vi "Send Software Trigger.vi"(8 "error in (no error)":errorcluster, 11 "VISA resource name":refnum<visa-resource-name>) -> (0 "error out":errorcluster, 3 "VISA resource name out":refnum<visa-resource-name>)   [LabVIEW 2015, in "Agilent 3352X Series.lvlib"]
doc: "Sends a software bus trigger to the instrument. You can use software bus triggers to trigger a frequency sweep. You must first set Trigger Source in the Configure Trigger VI to Software. \n\n<B>Note</B>:\n(1) Use this VI only with other low-level VIs. The high-level VIs automatically incorporate this functionality. \n(2) This VI does not check the instrument status. If you want to check the instrument status, call the Error Query VI at the conclusion of your sweep operation."
uses:
  Agilent 3352X Series.lvlib
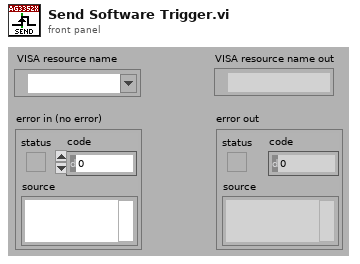
[diagram p1: front panel]
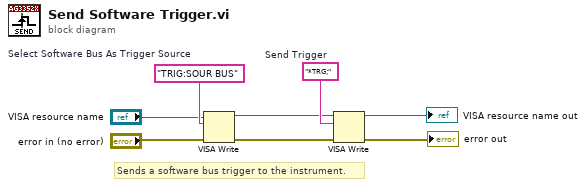
[diagram p0: block diagram]
diagram:
  w5 = "TRIG:SOUR BUS"  # Select Software Bus As Trigger Source
  w8 = "*TRG;"  # Send Trigger
  # "Sends a software bus trigger to the instrument."
  n1 = VISA Write(VISA resource name="VISA resource name", write buffer=w5, error in (no error)="error in (no error)") -> (VISA resource name out=w4:refnum<visa-resource-name>, error out=w1:errorcluster)  [unwired: 1 out]
  n2 = VISA Write(VISA resource name=w4, write buffer=w8, error in (no error)=w1) -> (VISA resource name out=→"VISA resource name out":refnum<visa-resource-name>, error out=→"error out":errorcluster)  [unwired: 1 out]
